vi "set variant name.vi"(8 "error in (no error)":errorcluster, 10 "new name":string, 11 "variant in":variant) -> (0 "error out":errorcluster, 3 "variant out":variant)   [LabVIEW 2017, in "JSON Value.lvclass"]
uses:
  JSON Value.lvclass
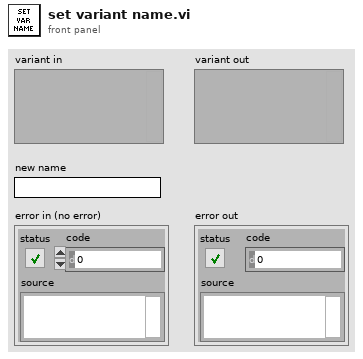
[diagram p1: front panel]
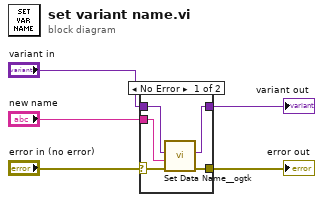
[diagram p0: block diagram]
diagram:
  n1 = case shown="No Error" "error in (no error)" {
    selector: "error in (no error)" -> [w8 w12]
    tunnel: "new name" -> [w9 _]
    tunnel: "variant in" -> [w10 w11]
    tunnel: [w7 w12] -> w2
    tunnel: [w6 w11] -> w1
    frame No Error {
      n2 = call "Set Data Name__ogtk.vi"("error in (no error)"=w8, "Data Name"=w9, "Data"=w10) -> ("error out"=w7:errorcluster, "Renamed Data"=w6:variant)  [unwired: 7 in]
    }
    frame Error {
    }
  }
  "error out" <- w2
  "variant out" <- w1
